vi "Compass Init.vi"(3 "Container State":T5, 4 "Previous State":variant, 5 "Previous Version":T4) -> (2 "Current State":T1={"Draw Options"={"Outer Border Color"=0, "Inner Border Color"=6316128, "Outer Gradient Color"=2565927, "Inner Gradient Color"=16860, "Compass North Pointer Color"=16711680, "Compass Pointer Color 1"=13355429, "Compass Pointer Color 2"=14934973, "Direction Pointer Color"=16765184, "Text Box Outline Color"=13355429, "Text Box Background Color"=14934973, "Scale Color"=16448250, "Text Color"=0, "Draw Gradient"=TRUE, "Draw Rose"=TRUE, "Simple Scale"=TRUE, "Draw Text"=FALSE, "Font Name"="Helvetica", "Angle Units"=enum."Degrees"}})   [LabVIEW 2017, in "Compass Indicator.xctl"]
uses:
  <vilib>/robotics/Controls/Compass Indicator/Compass Indicator.xctl
  <vilib>/_xctls/Container State.ctl
  <vilib>/robotics/Controls/Compass Indicator/_Compass Indicator Support Files/Compass State.ctl
  <vilib>/robotics/Controls/Compass Indicator/Compass Picture/Draw Options.ctl
  <vilib>/robotics/Controls/Utilities/Angle Units.ctl
  <vilib>/_xctls/Version.ctl
  <vilib>/robotics/Controls/Utilities/NI_Robotics_Control Utilities.lvlib
  <vilib>/_xctls/XControlSupport.lvlib
  <vilib>/robotics/Controls/Compass Indicator/Compass Picture/NI_Robotics_Compass Picture.lvlib
panel:
  in  "Default Indicator State":T1={"Draw Options"={"Outer Border Color"=0, "Inner Border Color"=6316128, "Outer Gradient Color"=2565927, "Inner Gradient Color"=16860, "Compass North Pointer Color"=16711680, "Compass Pointer Color 1"=13355429, "Compass Pointer Color 2"=14934973, "Direction Pointer Color"=16765184, "Text Box Outline Color"=13355429, "Text Box Background Color"=14934973, "Scale Color"=16448250, "Text Color"=0, "Draw Gradient"=TRUE, "Draw Rose"=TRUE, "Simple Scale"=TRUE, "Draw Text"=FALSE, "Font Name"="Helvetica", "Angle Units"=enum."Degrees"}}
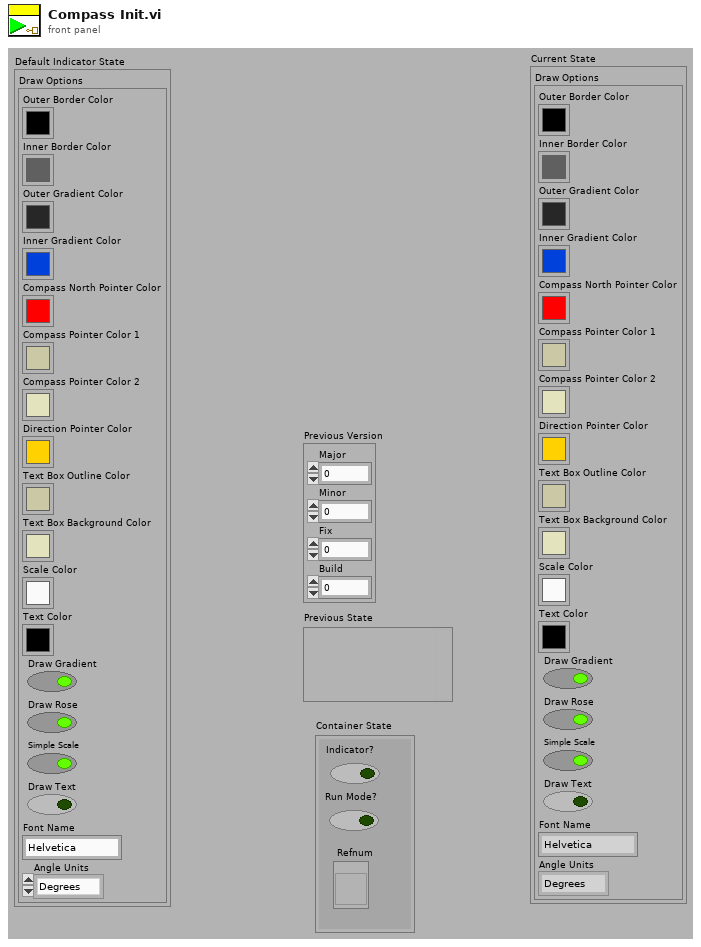
[diagram p1: front panel]
types:
  T1 = typedef "Compass Indicator.xctl/Compass State.ctl" = cluster{"Draw Options":T2}
  T2 = typedef "NI_Robotics_Compass Picture.lvlib/Draw Options.ctl" = cluster{"Outer Border Color":u32, "Inner Border Color":u32, "Outer Gradient Color":u32, "Inner Gradient Color":u32, "Compass North Pointer Color":u32, "Compass Pointer Color 1":u32, "Compass Pointer Color 2":u32, "Direction Pointer Color":u32, "Text Box Outline Color":u32, "Text Box Background Color":u32, "Scale Color":u32, "Text Color":u32, "Draw Gradient":bool, "Draw Rose":bool, "Simple Scale":bool, "Draw Text":bool, "Font Name":string, "Angle Units":T3}
  T3 = typedef "NI_Robotics_Control Utilities.lvlib/Angle Units.ctl" = enum16{"Radians", "Degrees"}
  T4 = typedef "XControlSupport.lvlib/Version.ctl" = cluster{"Major":u16, "Minor":u16, "Fix":u16, "Build":u16}
  T5 = typedef "XControlSupport.lvlib/Container State.ctl" = cluster{"Indicator?":bool, "Run Mode?":bool, " Refnum":refnum<vi>}
  T6 = cluster{"Draw Options":cluster{"Gradient?":bool, "Rose?":bool, "Simple Scale?":bool, "Text?":bool}, "Colors":cluster{"Outer Border Color":u32, "Inner Border Color":u32, "Outer Gradient Color":u32, "Inner Gradient Color":u32, "Compass North Pointer Color":u32, "Compass Pointer Color 1":u32, "Compass Pointer Color 2":u32, "Direction Pointer Color":u32, "Text Box Outline Color":u32, "Text Box Background Color":u32, "Scale Color":u32, "Text Color":u32}, "Font Name:":string}
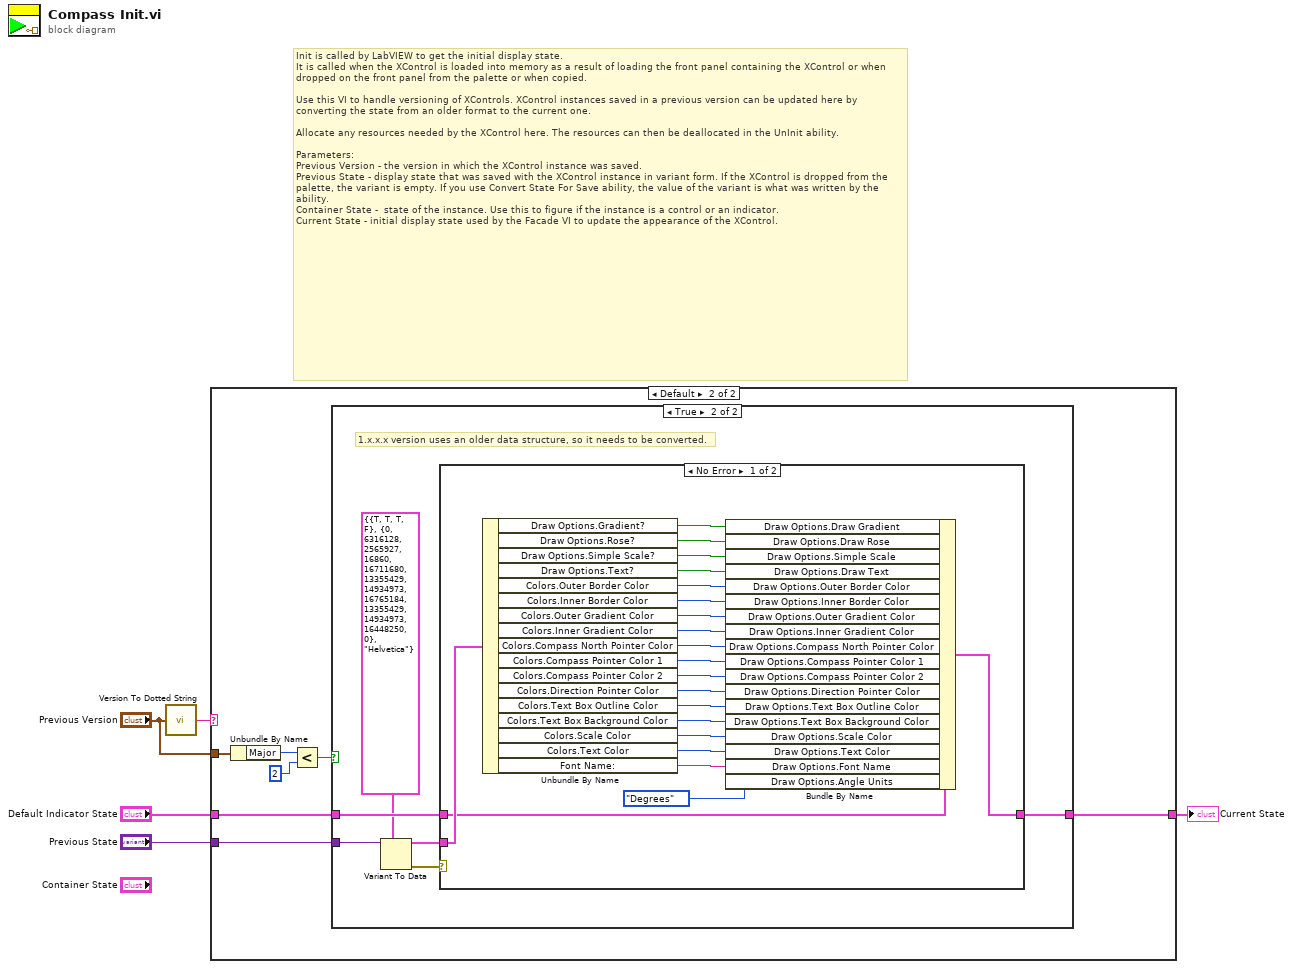
[diagram p0: block diagram]
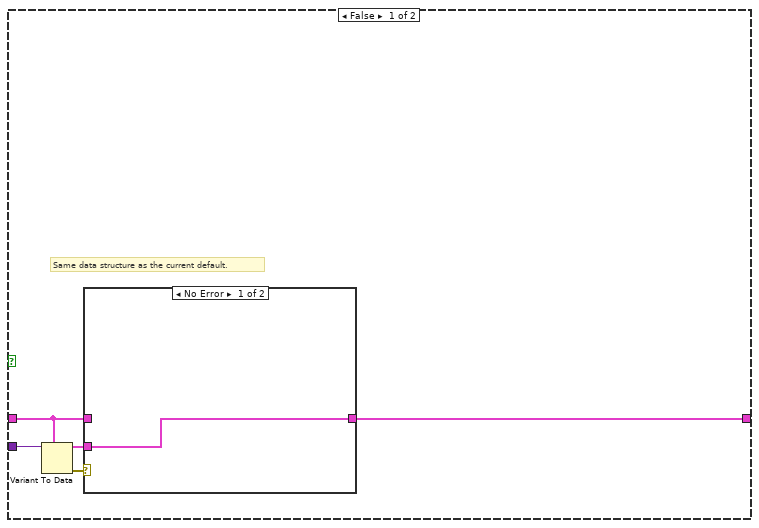
[diagram p3: hidden frame]
diagram:
  # "Init is called by LabVIEW to get the initial display state.\nIt is called when the XControl is loaded into memory as a result of loading the front panel containing the XControl or when dropped on the front panel from the palette or when copied.\n\nUse this VI to handle versioning of XControls. XControl instances saved in a previous version can be updated here by converting the state from an older format to the current one.\n\nAllocate any resources needed by the XControl here. The resources can then be deallocated in the UnInit ability.\n\nParameters:\nPrevious Version - the version in which the XControl instance was saved.\nPrevious State - display state that was saved with the XControl instance in variant form. If the XControl is dropped from the palette, the variant is empty. If you use Convert State For Save ability, the value of the variant is what was written by the ability. \nContainer State -  state of the instance. Use this to figure if the instance is a control or an indicator.\nCurrent State - initial display state used by the Facade VI to update the appearance of the XControl."
  n1 = call <vilib>:"Version To Dotted String.vi"("Version"="Previous Version") -> ("String Version"=w4:string)
  n2 = case shown="Default" w4 {
    tunnel: "Previous State" -> [_ w11]
    tunnel: [w6 w12] -> w2
    tunnel: "Default Indicator State" -> [w6 w13]
    tunnel: "Previous Version" -> [_ w10]
    frame "0.0.0.0" {
      # "Just created, use default state"
    }
    frame Default {
      n3 = Unbundle By Name(w10) -> ("Major"=w9:u16)
      n4 = Less?(x=w9, y=u16 2) -> (x < y?=w7:bool)
      n5 = case shown="True" w7 {
        tunnel: w13 -> [w16 w24]
        tunnel: [w15 w23] -> w12
        tunnel: w11 -> [w14 w22]
        frame False {
          # "Same data structure as the current default."
          n6 = Variant To Data(type=w16, Variant=w14) -> (data=w17:T1, error out=w18:errorcluster)  [unwired: 1 in]
          n7 = case shown="No Error" w18 {
            tunnel: w17 -> [w19 _]
            tunnel: [w19 w20] -> w15
            tunnel: w16 -> [_ w20]
            frame No Error {
            }
            frame Error {
              # "Error converting previously \nsaved state. Use default instead."
            }
          }
        }
        frame True {
          # "1.x.x.x version uses an older data structure, so it needs to be converted."
          n8 = Variant To Data(type=T6 {"Draw Options"={"Gradient?"=TRUE, "Rose?"=TRUE, "Simple Scale?"=TRUE, "Text?"=FALSE}, "Colors"={"Outer Border Color"=0, "Inner Border Color"=6316128, "Outer Gradient Color"=2565927, "Inner Gradient Color"=16860, "Compass North Pointer Color"=16711680, "Compass Pointer Color 1"=13355429, "Compass Pointer Color 2"=14934973, "Direction Pointer Color"=16765184, "Text Box Outline Color"=13355429, "Text Box Background Color"=14934973, "Scale Color"=16448250, "Text Color"=0}, "Font Name:"="Helvetica"} ("State"), Variant=w22) -> (data=w25:T6, error out=w26:errorcluster)  [unwired: 1 in]
          n9 = case shown="No Error" w26 {
            tunnel: w25 -> [w47 _]
            tunnel: [w45 w48] -> w23
            tunnel: w24 -> [w46 w48]
            frame No Error {
              n10 = Unbundle By Name(w47) -> ("Draw Options.Gradient?"=w44:bool, "Draw Options.Rose?"=w43:bool, "Draw Options.Simple Scale?"=w42:bool, "Draw Options.Text?"=w41:bool, "Colors.Outer Border Color"=w40:u32, "Colors.Inner Border Color"=w39:u32, "Colors.Outer Gradient Color"=w38:u32, "Colors.Inner Gradient Color"=w37:u32, "Colors.Compass North Pointer Color"=w36:u32, "Colors.Compass Pointer Color 1"=w35:u32, "Colors.Compass Pointer Color 2"=w34:u32, "Colors.Direction Pointer Color"=w33:u32, "Colors.Text Box Outline Color"=w32:u32, "Colors.Text Box Background Color"=w31:u32, "Colors.Scale Color"=w30:u32, "Colors.Text Color"=w29:u32, "Font Name:"=w28:string)
              n11 = Bundle By Name(cluster=w46, "Draw Options.Draw Gradient"=w44, "Draw Options.Draw Rose"=w43, "Draw Options.Simple Scale"=w42, "Draw Options.Draw Text"=w41, "Draw Options.Outer Border Color"=w40, "Draw Options.Inner Border Color"=w39, "Draw Options.Outer Gradient Color"=w38, "Draw Options.Inner Gradient Color"=w37, "Draw Options.Compass North Pointer Color"=w36, "Draw Options.Compass Pointer Color 1"=w35, "Draw Options.Compass Pointer Color 2"=w34, "Draw Options.Direction Pointer Color"=w33, "Draw Options.Text Box Outline Color"=w32, "Draw Options.Text Box Background Color"=w31, "Draw Options.Scale Color"=w30, "Draw Options.Text Color"=w29, "Draw Options.Font Name"=w28, "Draw Options.Angle Units"=Angle_Units."Degrees") -> (w45:T1)
            }
            frame Error {
              # "Error converting previously \nsaved state. Use default instead."
            }
          }
        }
      }
    }
  }
  "Current State" <- w2
